vi "Load TextConstant to md.vi"(8 "error in (no error)":errorcluster, 10 "Array":cluster{refnum<vi>, "Text":string}[](array[cluster]), 11 "Path":path) -> (0 "error out":errorcluster, 1 "logical AND":bool)   [LabVIEW 2014]
uses:
  JKI State Machine++.lvlib
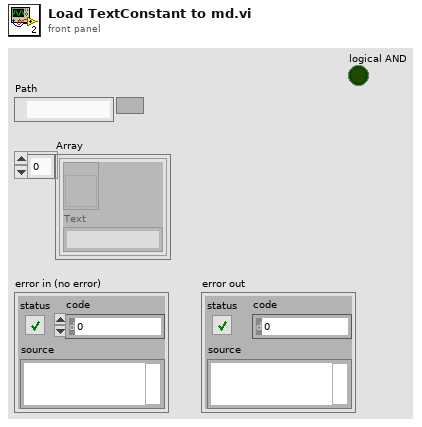
[diagram p1: front panel]
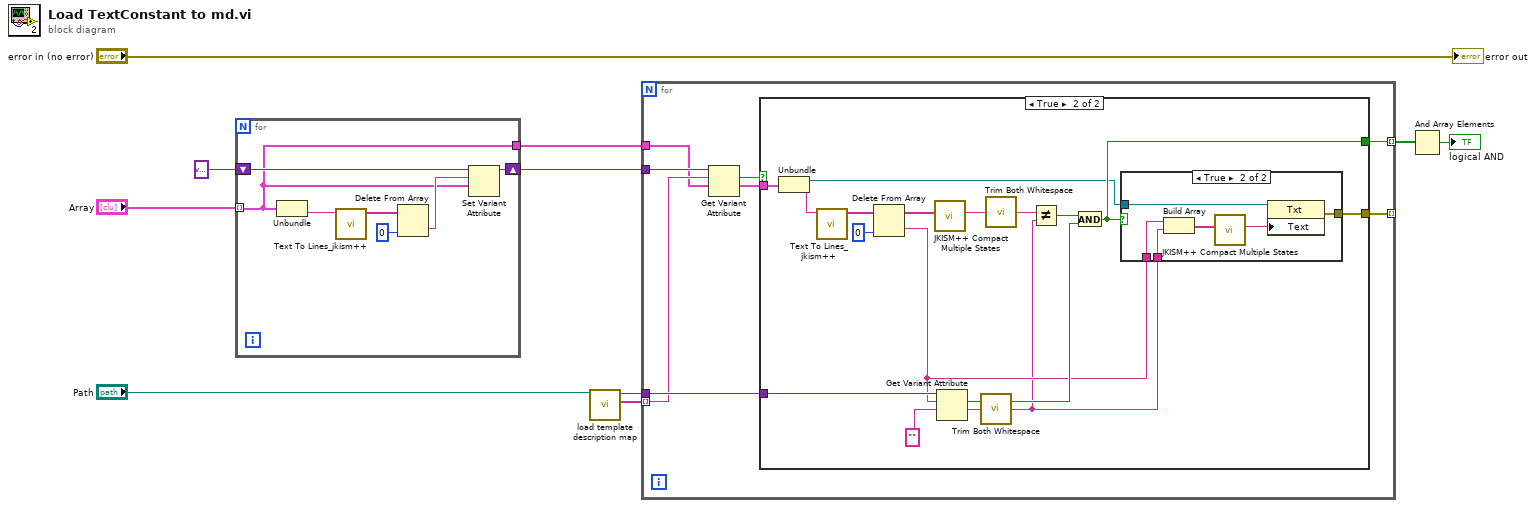
[diagram p0: block diagram]
diagram:
  n1 = for {
    tunnel: "Array" -> [w11] mode=indexing
    shift-right: [w14] -> w3
    shift-left: variant -> [w13]
    tunnel: [w11] -> w1
    n2 = Unbundle(w11) -> ("Text"=w17:string)  [unwired: 1 out]
    n3 = call "Text To Lines_jkism++.vi"("string"=w17) -> ("Lines"=w15:string[])  [unwired: 9 in, 1 out]
    n4 = Delete From Array(array=w15, index=0) -> (deleted portion=w12:string)  [unwired: 1 in, 1 out]
    n5 = Set Variant Attribute(Variant=w13, name=w12, value=w11) -> (Variant out=w14:variant)  [unwired: 1 in, 2 out]
  }
  n6 = call "load template description map.vi"("Path"="Path") -> ("Array"=w2:string[], "variant"=w9:variant)  [unwired: 8 in, 1 out]
  n7 = for {
    tunnel: [w24] -> w8 mode=indexing
    tunnel: [w23] -> _ mode=indexing
    tunnel: w3 -> [w22]
    tunnel: w2 -> [w21] mode=indexing
    tunnel: w1 -> [w20]
    tunnel: w9 -> [w25]
    n8 = Get Variant Attribute(Variant=w22, name=w21, default value (empty Variant)=w20) -> (found=w18:bool, value=w19:cluster{refnum<vi>, "Text":string})  [unwired: 1 in, 2 out]
    n9 = case shown="True" w18 {
      tunnel: w25 -> [_ w42]
      tunnel: [_ w33] -> w24
      tunnel: [_ w29] -> w23
      tunnel: w19 -> [_ w28]
      frame False {
      }
      frame True {
        n10 = Unbundle(w28) -> (w26:refnum<vi>, "Text"=w27:string)
        n11 = call "Text To Lines_jkism++.vi"("string"=w27) -> ("Lines"=w41:string[])  [unwired: 9 in, 1 out]
        n12 = Delete From Array(array=w41, index=0) -> (deleted portion=w32:string, array with subset deleted=w38:string[])  [unwired: 1 in]
        n13 = call "JKISM++ Compact Multiple States.vi"("States in Lines"=w38) -> ("States"=w37:string)  [unwired: 9 in]
        n14 = Get Variant Attribute(Variant=w42, name=w32, default value (empty Variant)="" ("deleted portion")) -> (found=w34:bool, value=w36:string)  [unwired: 1 in, 2 out]
        n15 = call "Trim Both Whitespace.vi"("string"=w36) -> ("trimmed string"=w31:string)  [unwired: 1 in]
        n16 = call "Trim Both Whitespace.vi"("string"=w37) -> ("trimmed string"=w30:string)  [unwired: 1 in]
        n17 = Not Equal?(x=w30, y=w31) -> (x != y?=w35:bool)
        n18 = And(x=w35, y=w34) -> (x .and. y?=w33:bool)
        n19 = case shown="True" w33 {
          tunnel: w26 -> [_ w48]
          tunnel: w31 -> [_ w47]
          tunnel: w32 -> [_ w44]
          tunnel: [_ w43] -> w29
          frame False {
          }
          frame True {
            n20 = Build Array(w44, w47) -> (w46:string[])
            n21 = call "JKISM++ Compact Multiple States.vi"("States in Lines"=w46) -> ("States"=w45:string)  [unwired: 9 in]
            n22 = property class="Txt"(reference=w48, "Text"=w45) -> (error out=w43:errorcluster)  [unwired: 1 in, 1 out]
          }
        }
      }
    }
  }
  n23 = And Array Elements(Boolean array=w8) -> (logical AND=→"logical AND":bool)
  "error out" <- "error in (no error)"
